vi "read_bytes.vi"(7 "read mode":T1(ring), 8 "error in (no error)":errorcluster, 9 "timeout (ms)":i32=-1, 10 "bytes to read":i32, 11 "TCP Connection in":refnum<class "TCP Connection.lvclass">) -> (0 "error out":errorcluster, 1 "data out":string, 2 "timeout?":bool, 3 "TCP Connection out":refnum<class "TCP Connection.lvclass">)   [LabVIEW 2019, in "TCP Connection.lvclass"]
uses:
  TCP Connection.lvclass
  TCP Connection.lvclass/TCP Connection.ctl
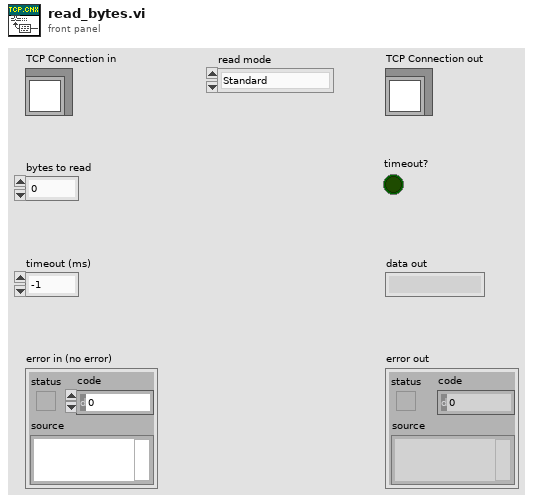
[diagram p1: front panel]
types:
  T1 = enum16{"Standard", "Buffered", "CRLF", "Immediate"}
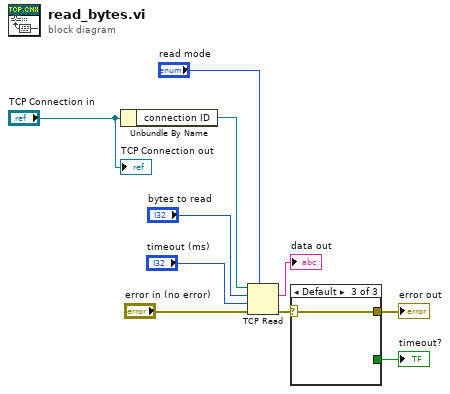
[diagram p0: block diagram]
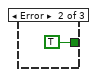
[diagram p3: hidden frame]
diagram:
  n1 = Unbundle By Name("TCP Connection in") -> ("connection ID"=w9:refnum<k5>)
  n2 = TCP Read(connection ID=w9, bytes to read="bytes to read", error in (no error)="error in (no error)", 7:"read mode", 9:"timeout (ms)") -> (data out=→"data out":string, error out=w3:errorcluster)  [unwired: 1 out]
  n3 = case shown="Default" w3 {
    selector: w3 -> [w11 _ w13]
    tunnel: [w11 _ w13] -> w2
    tunnel: [_ TRUE _] -> w1
    frame No Error {
    }
    frame Error {
    }
    frame Default {
    }
  }
  "error out" <- w2
  "timeout?" <- w1
  "TCP Connection out" <- "TCP Connection in"
